vi "ReadingMyAttribute.vi"(0 "reference in":refnum<class "MyG#Class.lvclass">, 5 "error in (no error)":errorcluster) -> (14 "reference out":refnum<class "MyG#Class.lvclass">, 16 "MyAttribute":dbl, 19 "error out":errorcluster)   [LabVIEW 2020, in "MyG#Class.lvclass"]
uses:
  MyG#Class.lvclass
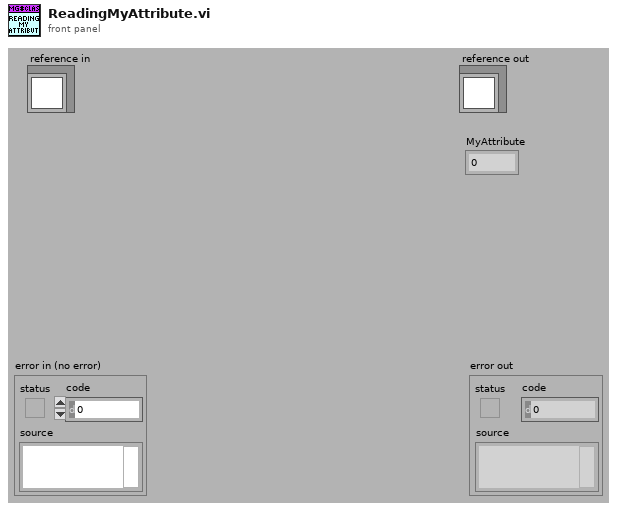
[diagram p1: front panel]
types:
  T1 = typedef "MyG#Class.lvclass/ObjectAttributes.ctl" = cluster{"MyAttribute":dbl}
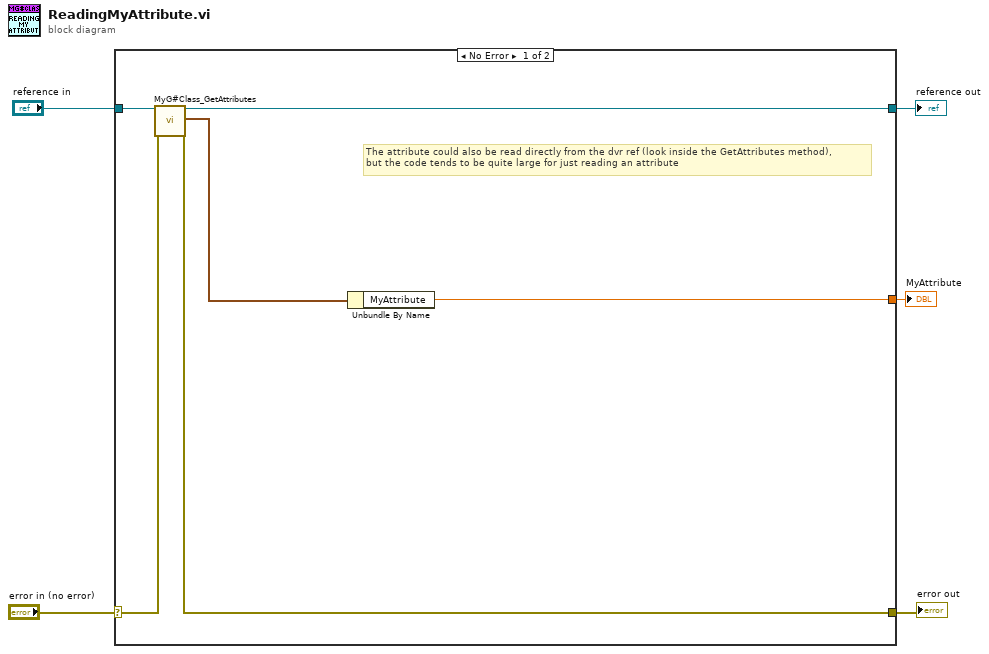
[diagram p0: block diagram]
diagram:
  n1 = case shown="No Error" "error in (no error)" {
    selector: "error in (no error)" -> [w11 w13]
    tunnel: [w9 w13] -> w4
    tunnel: [w6 w12] -> w2
    tunnel: "reference in" -> [w8 w12]
    tunnel: [w7 _] -> w1
    frame No Error {
      # "The attribute could also be read directly from the dvr ref (look inside the GetAttributes method),\nbut the code tends to be quite large for just reading an attribute"
      n2 = call "MyG#Class_GetAttributes.vi"("reference in"=w8, "error in (no error)"=w11) -> ("reference out"=w6:refnum<class "MyG#Class.lvclass">, "attributes"=w10:T1, "error out"=w9:errorcluster)  [unwired: 14 in, 1 out]
      n3 = Unbundle By Name(w10) -> ("MyAttribute"=w7:dbl)
    }
    frame Error {
    }
  }
  "error out" <- w4
  "reference out" <- w2
  "MyAttribute" <- w1
